vi "CC Calc Random Dither.vi"(8 "error in (no error)":errorcluster, 10 "Radius (arcsec)":dbl, 11 "RA and DEC":T1) -> (0 "error out":errorcluster, 3 "Dither RA and DEC":T1)   [LabVIEW 2021]
uses:
  typedefs/CC cluster RA and DEC.ctl
  <vilib>/numeric/Random Number (Range) DBL.vi
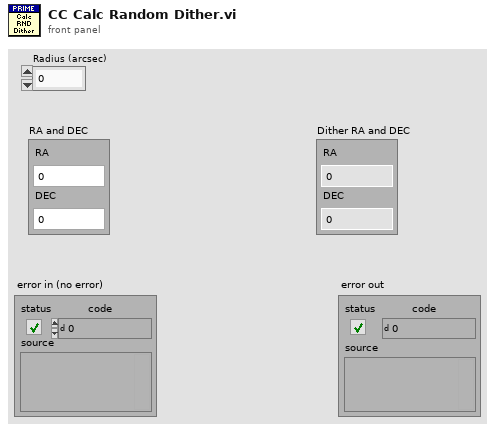
[diagram p1: front panel]
types:
  T1 = typedef "CC cluster RA and DEC.ctl" = cluster{"RA":dbl, "DEC":dbl}
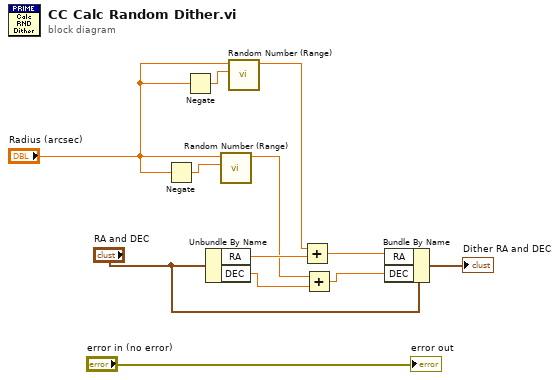
[diagram p0: block diagram]
diagram:
  n1 = Negate(x="Radius (arcsec)") -> (-x=w10:dbl)
  n2 = Negate(x="Radius (arcsec)") -> (-x=w11:dbl)
  n3 = Unbundle By Name("RA and DEC") -> ("RA"=w9:dbl, "DEC"=w7:dbl)
  n4 = call-poly <vilib>:"Random Number (Range).vi"("lower bound (0)"=w10, "upper bound (100)"="Radius (arcsec)") -> ("number"=w6:dbl)  [unwired: 9 in]
  n5 = call-poly <vilib>:"Random Number (Range).vi"("lower bound (0)"=w11, "upper bound (100)"="Radius (arcsec)") -> ("number"=w8:dbl)  [unwired: 9 in]
  n6 = Add(x=w8, y=w9) -> (x+y=w4:dbl)
  n7 = Add(x=w6, y=w7) -> (x+y=w3:dbl)
  n8 = Bundle By Name(cluster="RA and DEC", "RA"=w4, "DEC"=w3) -> (→"Dither RA and DEC":T1)
  "error out" <- "error in (no error)"
